vi "Boolean to Comms Status.vi"(11 "Comms":bool) -> (3 "GPS Status":u32)   [LabVIEW 2014]
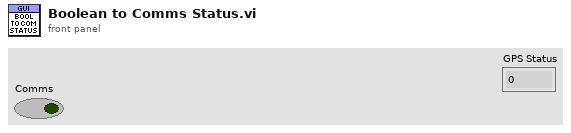
[diagram p1: front panel]
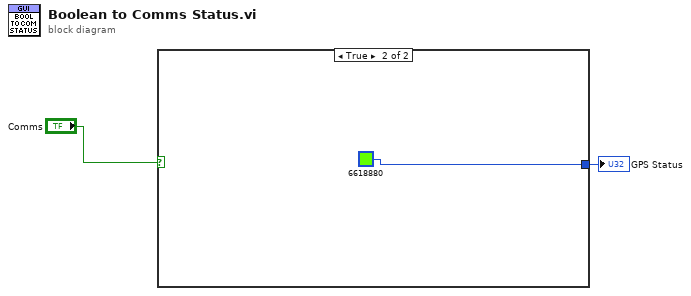
[diagram p0: block diagram]
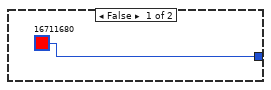
[diagram p2: hidden frame]
diagram:
  n1 = case shown="True" "Comms" {
    tunnel: [u32 16711680 u32 6618880] -> w1
    frame False {
    }
    frame True {
    }
  }
  "GPS Status" <- w1
